vi "Process.vi"(8 "error in":errorcluster, 11 "Inst.Magneto":refnum<class "Inst.Magneto.lvclass">) -> (0 "error out":errorcluster, 3 "Inst.Magneto out":refnum<class "Inst.Magneto.lvclass">)   [LabVIEW 2019, in "Inst.Magneto.lvclass"]
doc: "---------------------------------------------------------------\nJKI State Machine Objects™\nhttp://jki.net/state-machine-objects/\nCopyright (C) 2005-2015, JKI <info@jki.net>\nALL RIGHTS RESERVED"
uses:
  Inst.Magneto.lvclass
  C:/Program Files (x86)/National Instruments/LabVIEW 2019/vi.lib/JKI/JKI SMO/SMO/SMO.lvclass
  C:/Program Files (x86)/National Instruments/LabVIEW 2019/user.lib/LevyLab/Instrument Framework/SMOs/Instrument/Instrument.lvclass
  Typedefs/Inst.Magneto.Commands--Enum.ctl
  Typedefs/PrivateEvents--Inst.Magneto.MessageToProcess.ctl
  <userlib>/LevyLab/Instrument Framework/SMOs/RemoteControl/Typedefs/Message--Cluster.ctl
  <vilib>/JKI/JKI SMO/SMO/SMO.lvclass/SMO.ctl
  Inst.Magneto.lvclass/Inst.Magneto.ctl
  <vilib>/JKI/JKI SMO/SMO/Private/ReftoDVR--SMO.vi
  <userlib>/LevyLab/Instrument Framework/Instrument Types/VSource/Instrument.VSource.lvclass
  <vilib>/JKI/JKI SMO/SMO/SMO.lvclass
  <userlib>/LevyLab/Instrument Framework/SMOs/Instrument/Instrument.lvclass
  <userlib>/LevyLab/Instrument Framework/SMOs/RemoteControl/RemoteControl.lvclass
  <vilib>/httpClient/LabVIEWHTTPClient.lvlib
panel:
  out "Status":string
  out "State History":string
  # "Instrument.Magneto"
  # "Magneto"
  # "For instructions on how to use the JKI State Machine Objects, examples and video tutorials, visit:\nhttp://jki.net/state-machine-objects/\n\nJKI State Machine Objects™\nhttp://jki.net/state-machine-objects/\nCopyright (C) 2005-2015, JKI <info@jki.net>\nALL RIGHTS RESERVED"
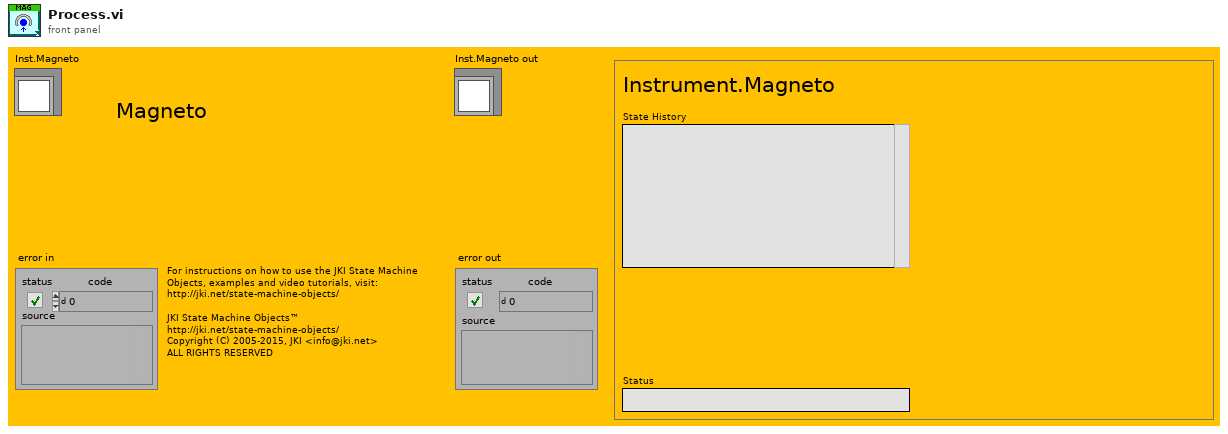
[diagram p1: front panel]
types:
  T1 = typedef "Inst.Magneto.lvclass/Inst.Magneto.Commands--Enum.ctl" = enum16{"GetRead", "Read", "Clear Values"}
  T2 = enum32{"invalid app kind", "Development System", "Run Time System", "Student Edition", "Embedded LabVIEW", "Evaluation", "Custom"}
  T3 = enum32{"Invalid", "Standard", "Closed", "Hidden", "Minimized", "Maximized"}
  T4 = typedef "RemoteControl.lvclass/Message--Cluster.ctl" = cluster{"Command":string, "Data":variant, "ID":string}
  T5 = typedef "Inst.Magneto.lvclass/PrivateEvents--Inst.Magneto.MessageToProcess.ctl" = cluster{"Message":T4}
  T6 = cluster{"Core":cluster{"Current VI Reference":refnum<vi>, "Close Panel on Exit?":bool, "Last Error":cluster{"error":errorcluster, "previous state":string, "remaining states":string}, "Shutdown?":bool}, "SelfRef":refnum<class "Inst.Magneto.lvclass">, "Running Step":i32, "sequence":string[], "MessageToProcess":T5}
  T7 = cluster{"Current VI Reference":refnum<vi>, "Close Panel on Exit?":bool, "Last Error":cluster{"error":errorcluster, "previous state":string, "remaining states":string}, "Shutdown?":bool}
  T8 = typedef "SMO.lvclass/Protected Events.ctl" = cluster{"StopProcesses":refnum<user-event>, "AbortProcesses":refnum<user-event>, "Config Changed":refnum<user-event>, "Dependency":refnum<user-event>}
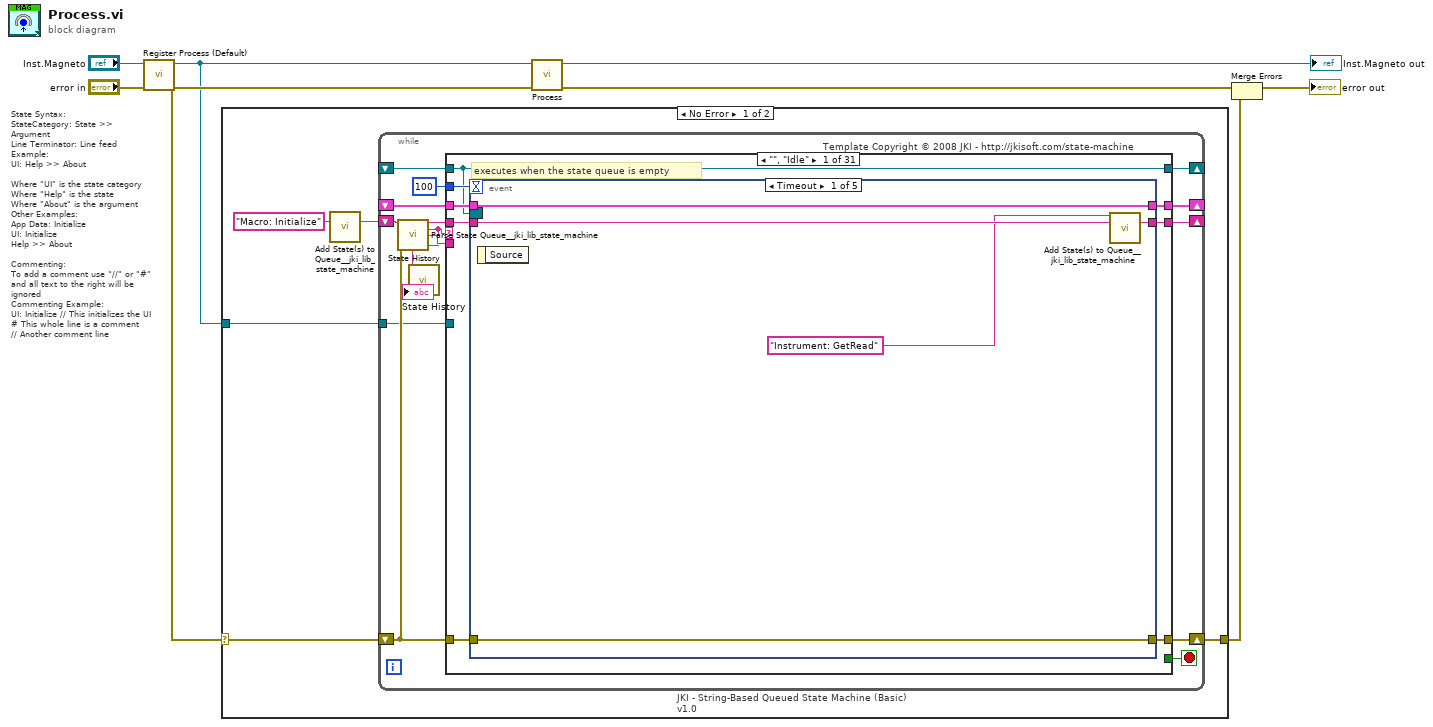
[diagram p0: block diagram]
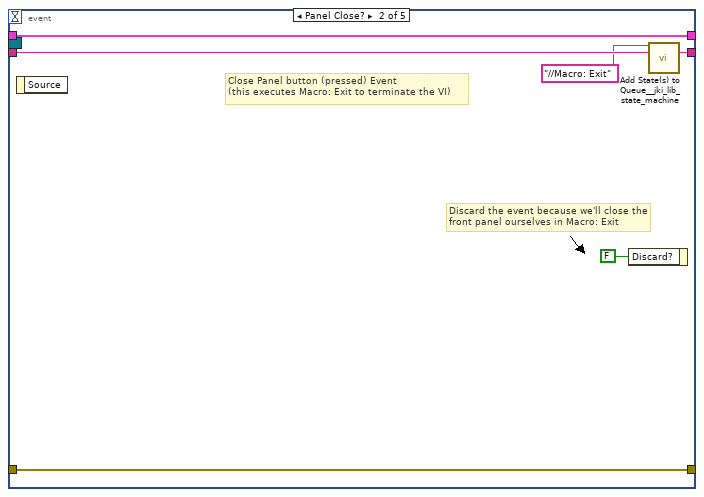
[diagram p2: hidden frame]
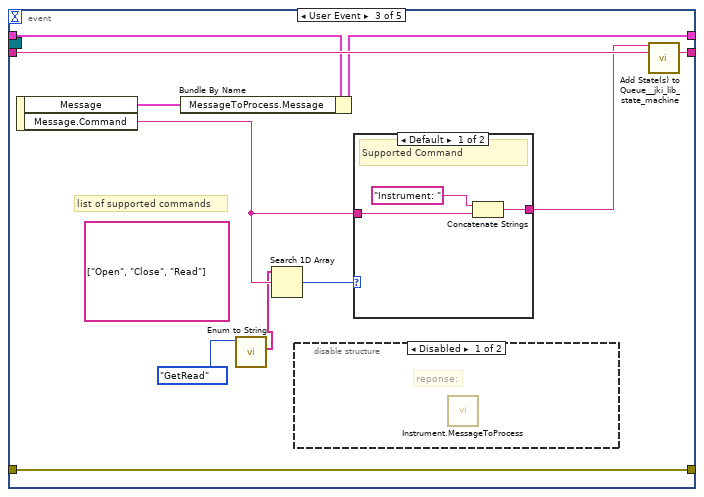
[diagram p3: hidden frame]
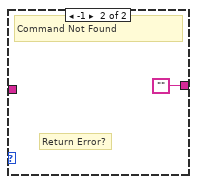
[diagram p5: hidden frame]
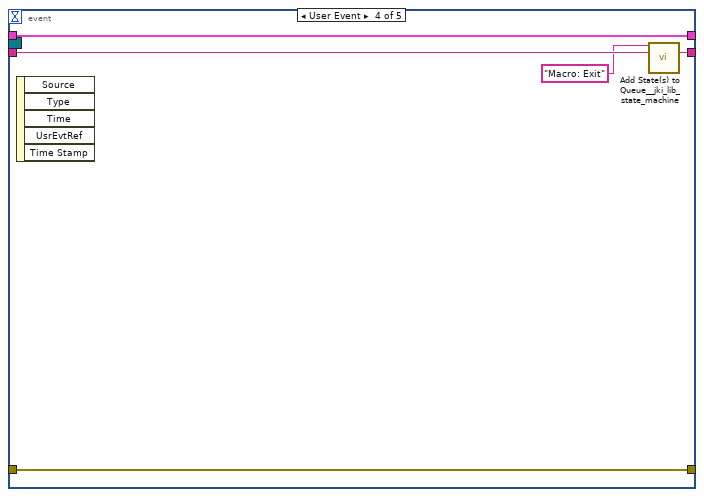
[diagram p6: hidden frame]
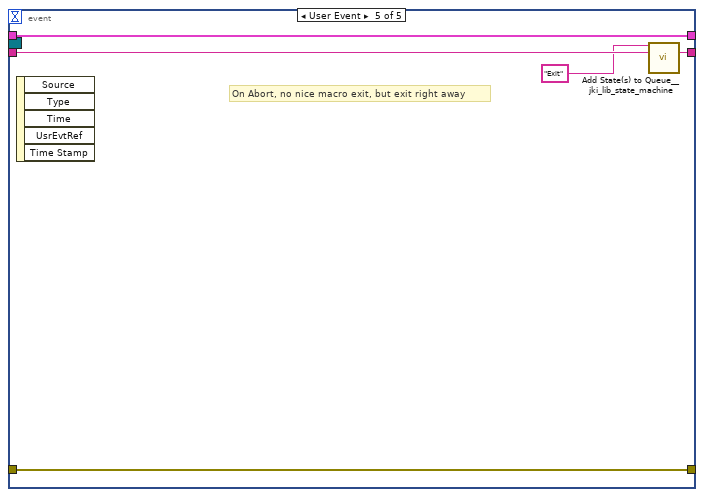
[diagram p7: hidden frame]
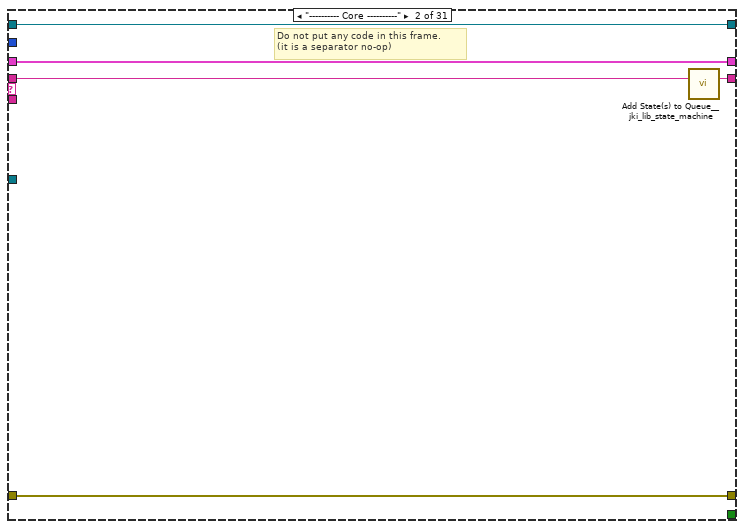
[diagram p8: hidden frame]
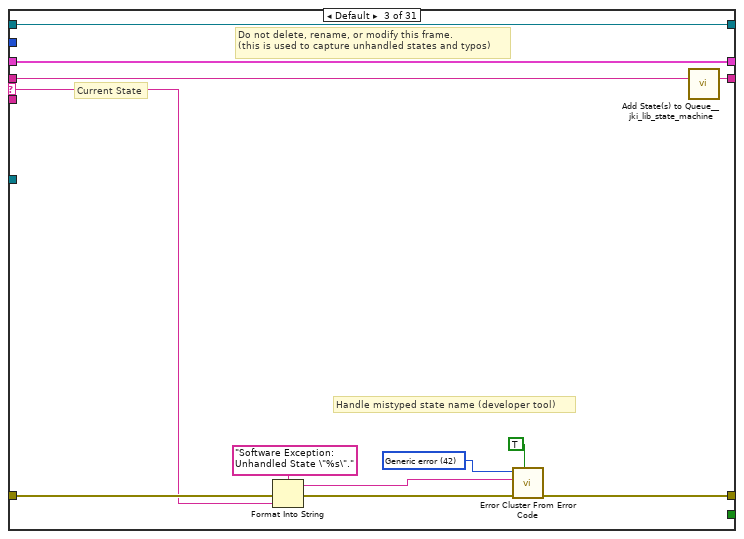
[diagram p9: hidden frame]
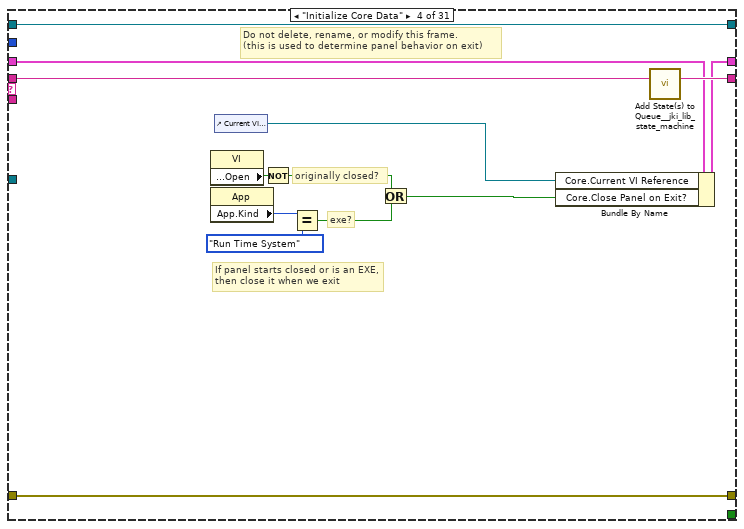
[diagram p10: hidden frame]
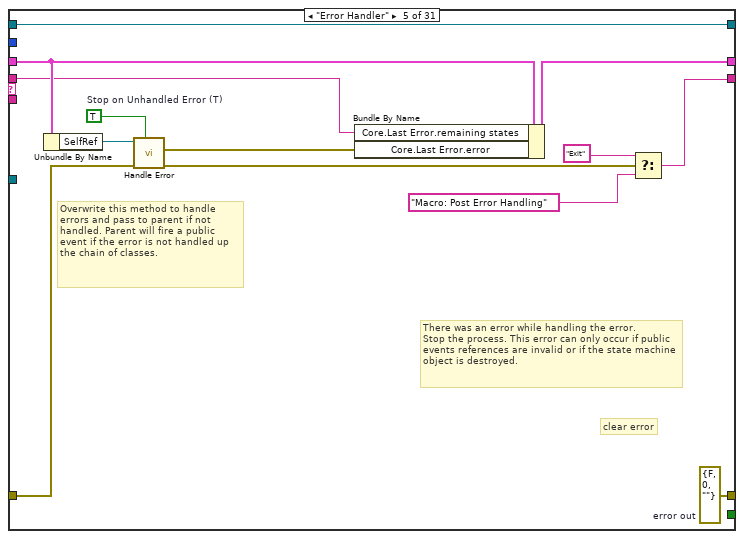
[diagram p11: hidden frame]
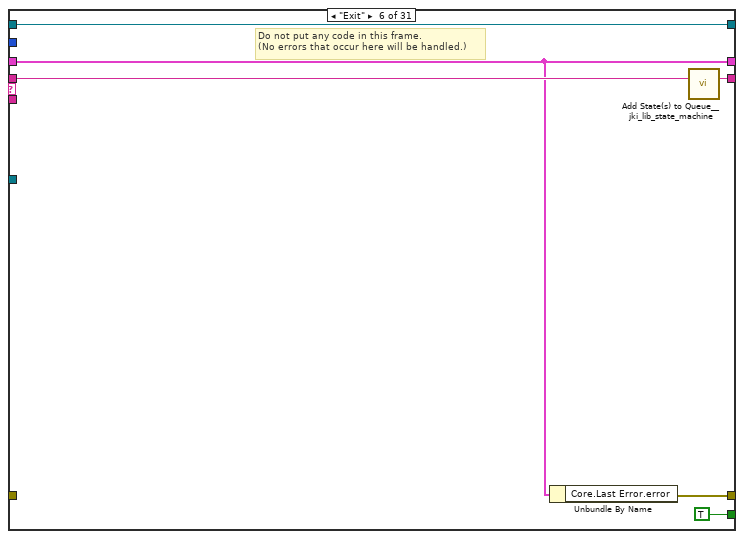
[diagram p12: hidden frame]
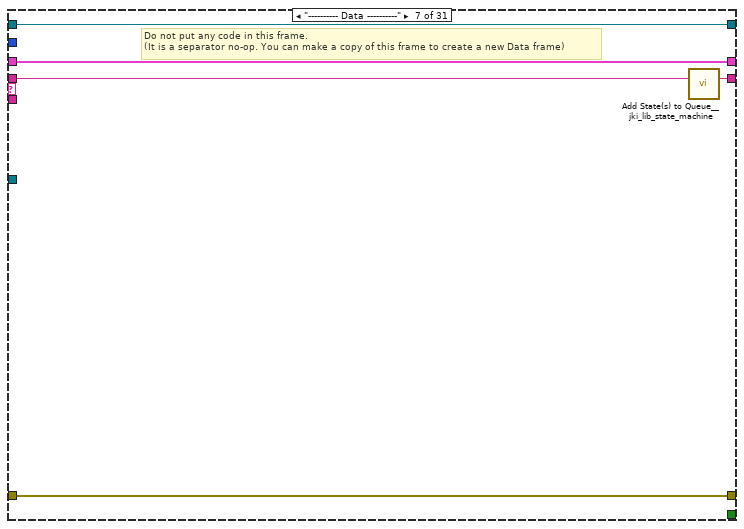
[diagram p13: hidden frame]
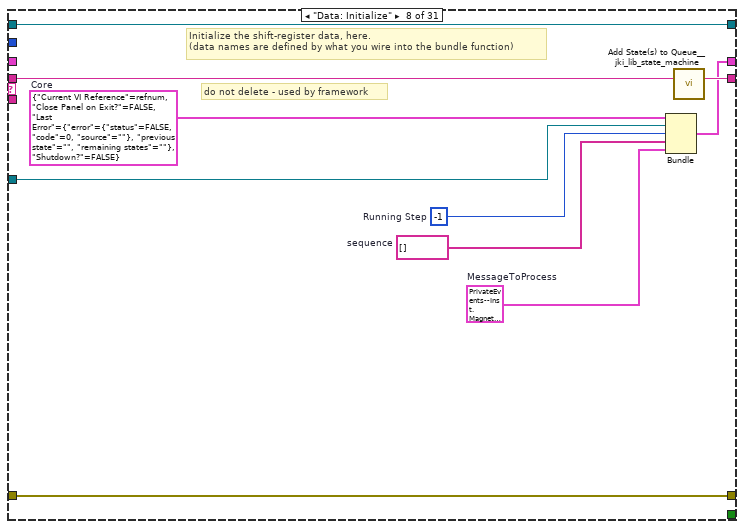
[diagram p14: hidden frame]
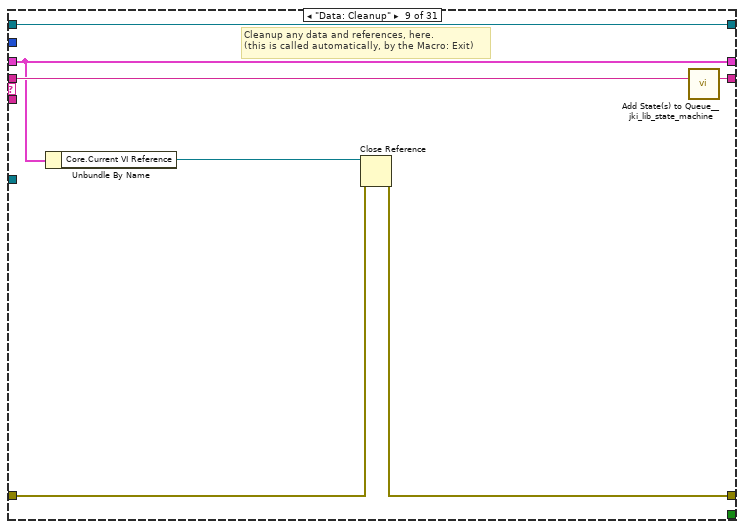
[diagram p15: hidden frame]
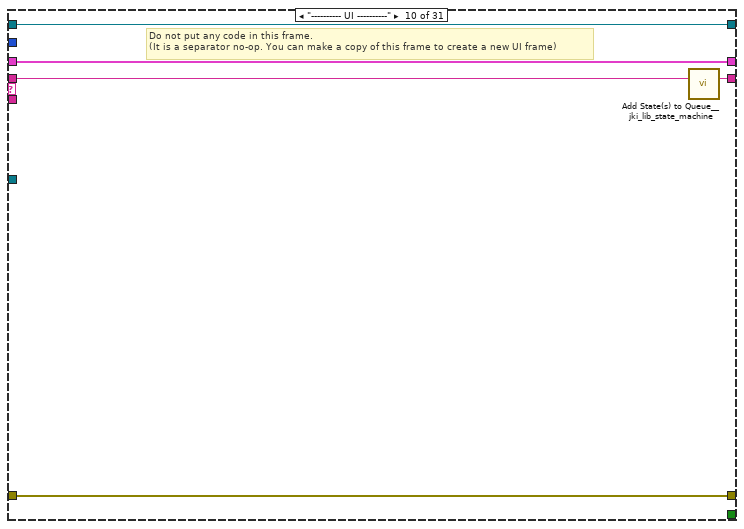
[diagram p16: hidden frame]
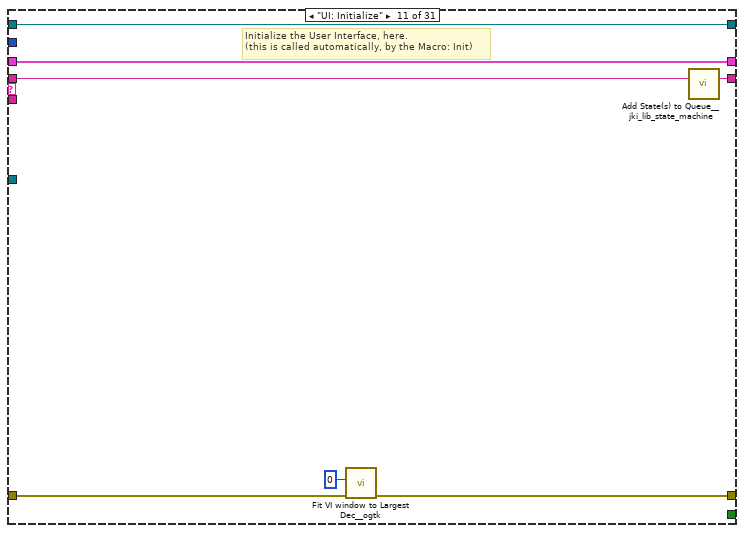
[diagram p17: hidden frame]
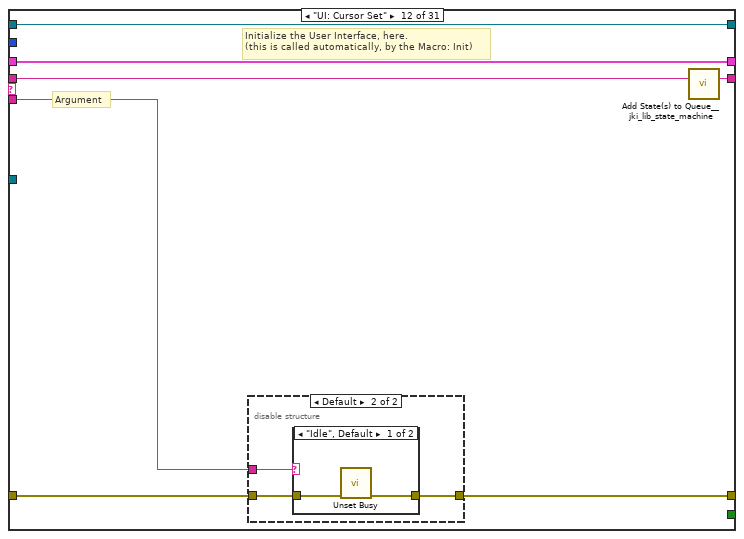
[diagram p18: hidden frame]
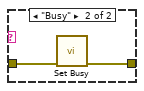
[diagram p20: hidden frame]
diagram:
  # "State Syntax:\nStateCategory: State >> Argument\nLine Terminator: Line feed\nExample:\nUI: Help >> About\n\nWhere \"UI\" is the state category\nWhere \"Help\" is the state\nWhere \"About\" is the argument\nOther Examples:\nApp Data: Initialize\nUI: Initialize\nHelp >> About\n\nCommenting:\nTo add a comment use \"//\" or \"#\" and all text to the right will be ignored\nCommenting Example:\nUI: Initialize // This initializes the UI\n# This whole line is a comment\n// Another comment line"
  n1 = call <vilib>:"Register Process (Default).vi"("error in (no error)"="error in", "SMO"="Inst.Magneto") -> ("error out"=w5:errorcluster, "SelfRef"=w4:refnum<class "Inst.Magneto.lvclass">)  [unwired: 8 in]
  n2 = case shown="No Error" w5 {
    selector: w5 -> [w10 w418]
    tunnel: w4 -> [w11 _]
    tunnel: [w9 w418] -> w1
    frame No Error {
      n3 = call <vilib>:"Add State(s) to Queue__jki_lib_state_machine.vi"("State(s) in (\"\")"="Macro: Initialize") -> ("States Out"=w13:string)  [unwired: 14 in]
      n4 = while "JKI - String-Based Queued State Machine (Basic) v1.0" {
        shift-right: [w22] -> _
        shift-left: _ -> [w21]
        shift-right: [w25] -> w9
        shift-left: w10 -> [w19]
        shift-right: [w24] -> _
        shift-left: w13 -> [w26]
        tunnel: w11 -> [w18]
        shift-right: [w17] -> _
        shift-left: _ -> [w16]
        stop <- w23 stop-if-true
        # "Template Copyright © 2008 JKI - http://jkisoft.com/state-machine"
        n5 = call <vilib>:"Parse State Queue__jki_lib_state_machine.vi"("State Queue"=w26, "Error In (no error)"=w19) -> ("Remaining States"=w28:string, "Current State"=w15:string, "Arguments"=w27:string)  [unwired: 11 in]
        n6 = call <userlib>:"State History.vi"("Current State"=w15) -> ("History"=→"State History":string)  [unwired: 10 in]
        n7 = case shown="\"\", \"Idle\"" w15 {
          selector: w15 -> [_ _ w79 _ _ _ _ _ _ _ _ _ _ _ _ _ _ _ _ _ _ _ _ _ _ _ _ _ _ _ _]
          tunnel: w28 -> [w36 w77 w83 w102 w107 w121 w126 w136 w143 w148 w155 w162 w178 w210 w229 w241 w262 w284 w289 w300 w305 w318 w324 w331 w340 w355 w364 w378 w392 w398 w417]
          tunnel: w27 -> [_ _ _ _ _ _ _ _ _ _ _ w156 w172 _ _ _ _ _ _ _ _ _ _ _ _ _ _ _ _ w393 w401]
          tunnel: w21 -> [w34 w74 w81 w93 w111 w117 w123 _ w138 w145 w153 w160 w174 w207 w226 w231 w252 w265 w286 w297 w302 w311 w322 w326 w336 w351 w360 w374 w388 w394 w407]
          tunnel: [w33 w75 w85 w99 w112 w116 w124 w128 w139 w146 w150 w157 w175 w208 w214 w239 w260 w267 w287 w291 w303 w314 w320 w328 w333 w349 w357 w369 w389 w395 w409] -> w25
          tunnel: w19 -> [w32 w75 w84 w99 w113 _ w124 w128 w140 w146 w149 w158 w176 w208 w218 w239 w260 w268 w287 w292 w303 w308 w320 w328 w332 w345 w356 w372 w389 w395 w403]
          tunnel: [w35 w76 w82 w101 w103 w120 w125 w135 w142 w147 w154 w161 w177 w209 w228 w240 w261 w283 w288 w299 w304 w317 w323 w330 w339 w354 w363 w377 w391 w397 w416] -> w24
          tunnel: [_ _ _ _ _ TRUE _ _ _ _ _ _ _ _ _ _ _ _ _ _ _ _ _ _ _ _ _ _ _ _ _] -> w23
          tunnel: [w31 w74 w81 w100 w110 w117 w123 w134 w138 w145 w153 w160 w174 w207 w226 w232 w253 w265 w286 w297 w302 w311 w322 w327 w337 w352 w361 w375 w388 w394 w406] -> w22
          tunnel: 100 ("Timeout") -> [w30 _ _ _ _ _ _ _ _ _ _ _ _ _ _ _ _ _ _ _ _ _ _ _ _ _ _ _ _ _ _]
          tunnel: w18 -> [_ _ _ _ _ _ _ w129 _ _ _ _ _ _ w222 _ _ w264 _ _ _ _ _ _ _ _ _ _ _ _ _]
          tunnel: [w29 w73 w78 w90 w115 w118 w122 w133 w137 w144 w152 w159 w171 w206 w227 w238 w259 w278 w285 w298 w301 w316 w321 w329 w338 w353 w362 w376 w390 w396 w415] -> w17
          tunnel: w16 -> [w29 w73 w78 w90 w115 w118 w122 w133 w137 w144 w152 w159 w171 w206 w227 w238 w259 w278 w285 w298 w301 _ w321 w329 w338 w353 w362 w376 w390 w396 w415]
          frame "", "Idle" {
            # "executes when the state queue is empty"
            n8 = event shown="[0] Timeout" {
              selector: w29 -> [_ _ _ _ _]
              dyn-events: _ -> [_ _ _ _ _]
              timeout: w30 -> [_ _ _ _ _]
              tunnel: w36 -> [w41 w47 w58 w67 w72]
              tunnel: [w40 w46 w57 w66 w71] -> w35
              tunnel: w34 -> [w38 w44 w51 w64 w69]
              tunnel: [w39 w45 w56 w65 w70] -> w33
              tunnel: w32 -> [w39 w45 w56 w65 w70]
              tunnel: [w38 w44 w52 w64 w69] -> w31
              event Timeout {
                n9 = event-data() -> ()  [unwired: 1 in, 1 out]
                n10 = call <vilib>:"Add State(s) to Queue__jki_lib_state_machine.vi"("State(s) in Front (\"\")"="Instrument: GetRead" ("State(s) in Front (\"\")"), "State(s) in (\"\")"=w41) -> ("States Out"=w40:string)  [unwired: 13 in]
              }
              event Panel Close? {
                # "Discard the event because we'll close the front panel ourselves in Macro: Exit"
                # "Close Panel button (pressed) Event\n(this executes Macro: Exit to terminate the VI)"
                n11 = event-data() -> ()  [unwired: 1 in, 1 out]
                n12 = event-data("Discard?"=FALSE) -> ()  [unwired: 1 in, 1 out]
                n13 = call <vilib>:"Add State(s) to Queue__jki_lib_state_machine.vi"("State(s) in Front (\"\")"="//Macro: Exit", "State(s) in (\"\")"=w47) -> ("States Out"=w46:string)  [unwired: 13 in]
              }
              event User Event {
                (unwired) string[] ["Open", "Close", "Read"]
                # "list of supported commands"
                n14 = event-data() -> ("Message"=w50:T4, "Message.Command"=w53:string)  [unwired: 1 in]
                n15 = Bundle By Name(cluster=w51, "MessageToProcess.Message"=w50) -> (w52:T6)
                n16 = call <userlib>:"Enum to String.vi"("Command"=Inst.Magneto.Commands--Enum."GetRead" ("Commands")) -> ("Commands []"=w48:string[])  [unwired: 9 in, 1 out]
                n17 = Search 1D Array(1D array=w48, element=w53) -> (index of element=w55:i32)  [unwired: 1 in]
                n18 = disable-structure shown="Disabled" {
                  frame Disabled {
                    # "reponse:"
                    n19 = call <userlib>:"Instrument.MessageToProcess.vi"() -> ()  [unwired: 10 in, 2 out]
                  }
                  frame Enabled {
                  }
                }
                n20 = case shown="Default" w55 {
                  tunnel: [w61 "" ("Empty String Constant")] -> w54
                  tunnel: w53 -> [w60 _]
                  frame Default {
                    # "Supported Command"
                    n21 = Concatenate Strings("Instrument: ", w60) -> (w61:string)
                  }
                  frame -1 {
                    # "Return Error?"
                    # "Command Not Found"
                  }
                }
                n22 = call <vilib>:"Add State(s) to Queue__jki_lib_state_machine.vi"("State(s) in Front (\"\")"=w54, "State(s) in (\"\")"=w58) -> ("States Out"=w57:string)  [unwired: 13 in]
              }
              event User Event {
                n23 = event-data() -> ()  [unwired: 1 in, 5 out]
                n24 = call <vilib>:"Add State(s) to Queue__jki_lib_state_machine.vi"("State(s) in Front (\"\")"="Macro: Exit", "State(s) in (\"\")"=w67) -> ("States Out"=w66:string)  [unwired: 13 in]
              }
              event User Event {
                # "On Abort, no nice macro exit, but exit right away"
                n25 = event-data() -> ()  [unwired: 1 in, 5 out]
                n26 = call <vilib>:"Add State(s) to Queue__jki_lib_state_machine.vi"("State(s) in Front (\"\")"="Exit", "State(s) in (\"\")"=w72) -> ("States Out"=w71:string)  [unwired: 13 in]
              }
            }
          }
          frame "---------- Core ----------" {
            # "Do not put any code in this frame.\n(it is a separator no-op)"
            n27 = call <vilib>:"Add State(s) to Queue__jki_lib_state_machine.vi"("State(s) in (\"\")"=w77) -> ("States Out"=w76:string)  [unwired: 14 in]
          }
          frame Default {
            w88 = 42 items=["No error", "Argument error", "Memory is full", "Out of zone", "End of file", "File already open", "Generic file I/O error", "File not found", "File permission error", "Disk is full", "Duplicate path", "Too many files open", "System feature not enabled", "Resource file not found", "Cannot add resource", "Resource not found", "Image not found", "Image memory error", "Pen does not exist", "Config type invalid", "Config token not found", "Config parse error", "Config memory error", "Bad external code format", "Bad external code offset", "External code not present", "Null window", "Destroy window error", "Null menu", "Print aborted", "Bad print record", "Print driver error", "Windows error during printing", "Memory error during printing", "Print dialog error", "Generic print error", "Invalid device refnum", "Device not found", "Device parameter error", "Device unit error", "Cannot open device", "Device call aborted", "Generic error", "Cancelled by user", "Object ID too low", "Object ID too high", "Object not in heap", "Unknown heap", "Unknown object (invalid DefProc)", "Unknown object (DefProc not in table)", "Message out of range", "Invalid (null) method", "Unknown message", "Manager call not supported", "Bad address", "Network operation in progress", "Network operation timed out", "Connection is busy", "Network attribute not supported", "Network error", "Address in use", "System out of memory", "Connection aborted", "Connection refused", "Not connected", "Already connected", "Connection closed", "Initialization error (interapplication manager)", "Bad occurrence", "Wait on unbound occurrence handler", "Occurrence queue overflow", "Datalog type conflict", "Unused", "Unrecognized type (interapplication manager)", "Memory corrupt", "Failed to make temporary DLL", "Old CIN version", "Drag socket not found", "Failed to load drop-object", "Failed to register OLE object", "Failed to release OLE object", "Format specifier type mismatch", "Unknown format specifier", "Too few format specifiers", "Too many format specifiers", "Scan failed", "Newer CIN version", "Error converting to variant", "Runtime menu error", "Password tampered", "Variant attribute not found", "Incompatible variant data type", "Event data is not available", "Event Store is not present", "Occurrence is not found", "Event Queue is not created", "Event info is not available", "Refnum passed is NULL", "Error retrieving Class GUID", "Error retrieving CoClass GUID", "Error retrieving TypeLib GUID.", "Bad built application magic bytes.", "Specific driver is different from the specific driver associated with the Logical Name.", "There is no session opened to the class driver.", "Max Error", "MAX - Error with config objects", "MAX - Error loading configuration", "MAX - Group not supported"]
            # "Current State"
            # "Do not delete, rename, or modify this frame.\n(this is used to capture unhandled states and typos)"
            # "Handle mistyped state name (developer tool)"
            n28 = Format Into String(format string="Software Exception: Unhandled State \"%s\"." ("message"), error in=w84, w79) -> (resulting string=w87:string, error out=w86:errorcluster)  [unwired: 1 in]
            n29 = call <vilib>:"Error Cluster From Error Code.vi"("show call chain? (False)"=TRUE, "error in (no error)"=w86, "error message (\"\")"=w87, "error code (0)"=w88) -> ("error out"=w85:errorcluster)  [unwired: 5 in]
            n30 = call <vilib>:"Add State(s) to Queue__jki_lib_state_machine.vi"("State(s) in (\"\")"=w83) -> ("States Out"=w82:string)  [unwired: 14 in]
          }
          frame "Initialize Core Data" {
            # "Do not delete, rename, or modify this frame.\n(this is used to determine panel behavior on exit)"
            # "originally closed?"
            # "exe?"
            # "If panel starts closed or is an EXE, then close it when we exit"
            n31 = property class="VI"() -> ("Front Panel.Open"=w98:bool)  [unwired: 2 in, 2 out]
            n32 = property class="App"() -> ("App.Kind"=w97:T2)  [unwired: 2 in, 2 out]
            n33 = control-ref of="Current VI Reference"() -> (w91:refnum<vi>)
            n34 = Not(x=w98) -> (.not. x?=w95:bool)
            n35 = Equal?(x=w97, y=T2."Run Time System" ("Application:Kind")) -> (x = y?=w94:bool)
            n36 = Or(x=w95, y=w94) -> (x .or. y?=w92:bool)
            n37 = Bundle By Name(cluster=w93, "Core.Current VI Reference"=w91, "Core.Close Panel on Exit?"=w92) -> (w100:T6)
            n38 = call <vilib>:"Add State(s) to Queue__jki_lib_state_machine.vi"("State(s) in (\"\")"=w102) -> ("States Out"=w101:string)  [unwired: 14 in]
          }
          frame "Error Handler" {
            w108 = TRUE  # Stop on Unhandled Error (T)
            w112 = errorcluster {"status"=FALSE, "code"=0, "source"=""}  # error out
            # "clear error"
            # "There was an error while handling the error.\nStop the process. This error can only occur if public events references are invalid or if the state machine object is destroyed."
            # "Overwrite this method to handle errors and pass to parent if not handled. Parent will fire a public event if the error is not handled up the chain of classes."
            n39 = Unbundle By Name(w111) -> ("SelfRef"=w114:refnum<class "Inst.Magneto.lvclass">)
            n40 = call-dynamic "Handle Error.vi"("Stop on Unhandled Error (T)"=w108, "error in"=w113, "SMO"=w114) -> ("handling error"=w104:errorcluster, "Unhandled error"=w109:errorcluster)  [unwired: 6 in, 1 out]
            n41 = Bundle By Name(cluster=w111, "Core.Last Error.remaining states"=w107, "Core.Last Error.error"=w109) -> (w110:T6)
            n42 = Select(t="Exit", s=w104, f="Macro: Post Error Handling") -> (s? t:f=w103:string)
          }
          frame "Exit" {
            # "Do not put any code in this frame.\n(No errors that occur here will be handled.)"
            n43 = Unbundle By Name(w117) -> ("Core.Last Error.error"=w116:errorcluster)
            n44 = call <vilib>:"Add State(s) to Queue__jki_lib_state_machine.vi"("State(s) in (\"\")"=w121) -> ("States Out"=w120:string)  [unwired: 14 in]
          }
          frame "---------- Data ----------" {
            # "Do not put any code in this frame.\n(It is a separator no-op. You can make a copy of this frame to create a new Data frame)"
            n45 = call <vilib>:"Add State(s) to Queue__jki_lib_state_machine.vi"("State(s) in (\"\")"=w126) -> ("States Out"=w125:string)  [unwired: 14 in]
          }
          frame "Data: Initialize" {
            w127 = T5 {"Message"={"Command"="", "Data"=variant(string ""), "ID"=""}}  # MessageToProcess
            w130 = string[] []  # sequence
            w131 = -1  # Running Step
            w132 = T7 {"Current VI Reference"=refnum, "Close Panel on Exit?"=FALSE, "Last Error"={"error"={"status"=FALSE, "code"=0, "source"=""}, "previous state"="", "remaining states"=""}, "Shutdown?"=FALSE}  # Core
            # "do not delete - used by framework"
            # "Initialize the shift-register data, here.\n(data names are defined by what you wire into the bundle function)"
            n46 = Bundle("Core"=w132, "SelfRef"=w129, "Running Step"=w131, "sequence"=w130, "MessageToProcess"=w127) -> (w134:T6)  [unwired: 1 in]
            n47 = call <vilib>:"Add State(s) to Queue__jki_lib_state_machine.vi"("State(s) in (\"\")"=w136) -> ("States Out"=w135:string)  [unwired: 14 in]
          }
          frame "Data: Cleanup" {
            # "Cleanup any data and references, here.\n(this is called automatically, by the Macro: Exit)"
            n48 = Unbundle By Name(w138) -> ("Core.Current VI Reference"=w141:refnum<vi>)
            n49 = Close Reference(reference=w141, error in (no error)=w140) -> (error out=w139:errorcluster)
            n50 = call <vilib>:"Add State(s) to Queue__jki_lib_state_machine.vi"("State(s) in (\"\")"=w143) -> ("States Out"=w142:string)  [unwired: 14 in]
          }
          frame "---------- UI ----------" {
            # "Do not put any code in this frame.\n(It is a separator no-op. You can make a copy of this frame to create a new UI frame)"
            n51 = call <vilib>:"Add State(s) to Queue__jki_lib_state_machine.vi"("State(s) in (\"\")"=w148) -> ("States Out"=w147:string)  [unwired: 14 in]
          }
          frame "UI: Initialize" {
            # "Initialize the User Interface, here.\n(this is called automatically, by the Macro: Init)"
            n52 = call <userlib>:"Fit VI window to Largest Dec__ogtk.vi"("error in (no error)"=w149, "border spacing (2 px)"=0) -> ("error out"=w150:errorcluster)  [unwired: 4 in, 1 out]
            n53 = call <vilib>:"Add State(s) to Queue__jki_lib_state_machine.vi"("State(s) in (\"\")"=w155) -> ("States Out"=w154:string)  [unwired: 14 in]
          }
          frame "UI: Cursor Set" {
            # "Argument"
            # "Initialize the User Interface, here.\n(this is called automatically, by the Macro: Init)"
            n54 = disable-structure shown="Default" {
              disable-tunnel: w158 -> [w163 w166]
              disable-tunnel: [w163 w165] -> w157
              disable-tunnel: w156 -> [_ w164]
              frame condition #0 {
              }
              frame condition #1 (active) {
                n55 = case shown="\"Idle\", Default" w164 {
                  tunnel: w166 -> [w168 w170]
                  tunnel: [w167 w169] -> w165
                  frame "Idle", Default {
                    n56 = call <vilib>:"Unset Busy.vi"("error in (no error)"=w168) -> ("error out"=w167:errorcluster)  [unwired: 10 in]
                  }
                  frame "Busy" {
                    n57 = call <vilib>:"Set Busy.vi"("error in (no error)"=w170) -> ("error out"=w169:errorcluster)  [unwired: 9 in, 1 out]
                  }
                }
              }
            }
            n58 = call <vilib>:"Add State(s) to Queue__jki_lib_state_machine.vi"("State(s) in (\"\")"=w162) -> ("States Out"=w161:string)  [unwired: 14 in]
          }
          frame "UI: Front Panel State" {
            # "Argument"
            # "Set Front Panel Open or Closed\n(Usage: \"UI: Front Panel State >> Open|Close\")"
            n59 = Unbundle By Name(w174) -> ("Core.Current VI Reference"=w173:refnum<vi>)
            n60 = disable-structure shown="Default" {
              disable-tunnel: w176 -> [w182 w205]
              disable-tunnel: [w181 w205] -> w175
              disable-tunnel: w173 -> [w180 _]
              disable-tunnel: w172 -> [w179 _]
              frame condition #0 (active) {
                n61 = case shown="\"Close\"" w179 {
                  tunnel: w182 -> [w186 w199]
                  tunnel: [w188 w200] -> w181
                  tunnel: w180 -> [w187 w197]
                  frame "Open", Default {
                    n62 = property class="VI"(reference=w187, error in=w186) -> (reference out=w184:refnum<vi>, error out=w185:errorcluster, "FP.State"=w183:T3)
                    n63 = case shown="\"Closed\"" w183 {
                      tunnel: [w191 w194] -> w188
                      tunnel: w185 -> [w190 w194]
                      tunnel: w184 -> [w189 _]
                      frame "Closed" {
                        n64 = invoke class="VI" method="FP.Open"(reference=w189, error in=w190, "Activate"=TRUE, "State"=T3."Standard") -> (error out=w191:errorcluster)  [unwired: 1 in, 4 out]
                      }
                      frame Default {
                      }
                    }
                  }
                  frame "Close" {
                    n65 = property class="VI"(reference=w197, error in=w199) -> (reference out=w196:refnum<vi>, error out=w198:errorcluster, "FP.State"=w195:T3)
                    n66 = case shown="Default" w195 {
                      tunnel: [w201 w204] -> w200
                      tunnel: w198 -> [w201 w203]
                      tunnel: w196 -> [_ w202]
                      frame "Invalid", "Closed" {
                      }
                      frame Default {
                        n67 = invoke class="VI" method="FP.Close"(reference=w202, error in=w203) -> (error out=w204:errorcluster)  [unwired: 1 in, 2 out]
                      }
                    }
                  }
                }
              }
              frame condition #1 {
              }
            }
            n68 = call <vilib>:"Add State(s) to Queue__jki_lib_state_machine.vi"("State(s) in (\"\")"=w178) -> ("States Out"=w177:string)  [unwired: 14 in]
          }
          frame "---------- Macro ----------" {
            # "Do not put any code in this frame.\n(It is a separator no-op. You can make a copy of this frame to create a new Macro frame)"
            n69 = call <vilib>:"Add State(s) to Queue__jki_lib_state_machine.vi"("State(s) in (\"\")"=w210) -> ("States Out"=w209:string)  [unwired: 14 in]
          }
          frame "Macro: Initialize" {
            # "Initialization Macro\n(This is called once, when the VI starts)"
            n70 = call-dynamic "Read Debug Mode.vi"("error in (no error)"=w218, "Instrument in"=w222) -> ("error out"=w217:errorcluster, "Debug Mode?"=w219:bool)  [unwired: 7 in, 1 out]
            n71 = call <userlib>:"Wait (ms)__ogtk.vi"("error in (no error)"=w217, "milliseconds to wait"=u32 0) -> ("error out"=w214:errorcluster)  [unwired: 8 in, 1 out]
            n72 = Select(t="Open", s=w219, f="Close") -> (s? t:f=w215:string)
            n73 = Format Into String(format string="UI: Initialize\nUI: Front Panel State >> %s\nInstrument: Open Hardware", initial string="", w215) -> (resulting string=w216:string)  [unwired: 1 in, 1 out]
            n74 = call <vilib>:"Add State(s) to Queue__jki_lib_state_machine.vi"("State(s) in Front (\"\")"="Data: Initialize\nInitialize Core Data\nEvents: Register", "State(s) in (\"\")"="Process: Sync", "State(s) at Back (\"\")"=w216) -> ("States Out"=w224:string)  [unwired: 12 in]
            n75 = call <vilib>:"Add State(s) to Queue__jki_lib_state_machine.vi"("State(s) in Front (\"\")"=w224, "State(s) in (\"\")"=w229) -> ("States Out"=w228:string)  [unwired: 13 in]
          }
          frame "Macro: Post Error Handling" {
            # "Clear Last Error?"
            n76 = Unbundle By Name(w231) -> ("Core.Last Error.remaining states"=w233:string, "Core.Shutdown?"=w234:bool)
            n77 = Unbundle By Name(w231) -> ("Core.Last Error.error"=w237:errorcluster)
            n78 = case shown="False" FALSE {
              tunnel: w237 -> [w245 _]
              tunnel: [w245 _] -> w236
              frame False {
              }
              frame True {
              }
            }
            n79 = case shown="True" w234 {
              tunnel: w233 -> [w242 w244]
              tunnel: [w242 w243] -> w230
              frame False {
                # "These are the remaining states (at the moment the error occured). States can be altered according to business logic."
                # "NOT SHUTTING DOWN"
              }
              frame True {
                # "Developer can decide to alter the states but should be aware that during the shutdown process, there are certain states that must be run for the SMO to properly shut itself (and this process) down. As such, one can add states to perform additional clean-ups, but should append the remaining state to be executed."
                # "SHUTTING DOWN"
                n80 = call <vilib>:"Add State(s) to Queue__jki_lib_state_machine.vi"("State(s) in (\"\")"=w244) -> ("States Out"=w243:string)  [unwired: 14 in]
              }
            }
            n81 = Bundle By Name(cluster=w231, "Core.Last Error.error"=w236) -> (w232:T6)
            n82 = call <vilib>:"Add State(s) to Queue__jki_lib_state_machine.vi"("State(s) in Front (\"\")"=w230, "State(s) in (\"\")"=w241) -> ("States Out"=w240:string)  [unwired: 13 in]
          }
          frame "Macro: Run Sequence" {
            # "0,1,2,3,4,"
            # "5"
            # "Do not put any code in this frame.\n(It is a separator no-op. You can make a copy of this frame to create a new Macro frame)"
            n83 = Unbundle By Name(w252) -> ("sequence"=w248:string[], "Running Step"=w246:i32)
            n84 = Array Size(array=w248) -> (size(s)=w258:i32)
            n85 = Index Array(array=w248, index=w246) -> (element=w247:string)
            n86 = Greater Or Equal?(x=w258, y=w246) -> (x >= y?=w250:bool)
            n87 = Select(t=-1 ("Running Step"), s=w250, f=w246) -> (s? t:f=w257:i32)
            n88 = Bundle By Name(cluster=w252, "Running Step"=w257) -> (w253:T6)
            n89 = Select(t="Sequence: Status >> ...", s=w250, f="Idle //Check Event Structure\nMacro: Run Sequence" ("State(s) at Back (\"\")")) -> (s? t:f=w249:string)
            n90 = call <vilib>:"Add State(s) to Queue__jki_lib_state_machine.vi"("State(s) in Front (\"\")"=w247, "State(s) at Back (\"\")"=w249) -> ("States Out"=w251:string)  [unwired: 13 in]
            n91 = call <vilib>:"Add State(s) to Queue__jki_lib_state_machine.vi"("State(s) in Front (\"\")"=w251, "State(s) in (\"\")"=w262) -> ("States Out"=w261:string)  [unwired: 13 in]
          }
          frame "Macro: Exit" {
            # "Exit Macro\n(This is called once, when the VI exits)"
            n92 = Unbundle By Name(w265) -> ("Core.Close Panel on Exit?"=w282:bool)
            n93 = call-dynamic "Read Debug Mode.vi"("error in (no error)"=w268, "Instrument in"=w264) -> ("error out"=w267:errorcluster, "Debug Mode?"=w266:bool)  [unwired: 7 in, 1 out]
            n94 = Select(t="Open", s=w266, f="Close") -> (s? t:f=w272:string)
            n95 = call <vilib>:"Build State String with Arguments__JKI_lib_State_Machine.vi"("Arguments (\"\")"=w272, "State"="UI: Front Panel State") -> ("State with Arguments"=w269:string)  [unwired: 4 in]
            n96 = Select(t=w269, s=w282, f="" ("Empty String Constant")) -> (s? t:f=w280:string)
            n97 = call <vilib>:"Add State(s) to Queue__jki_lib_state_machine.vi"("State(s) in Front (\"\")"="Data: Cleanup\nEvents: Unregister", "State(s) in (\"\")"="Process: Sync", "State(s) at Back (\"\")"="Exit") -> ("States Out"=w275:string)  [unwired: 12 in]
            n98 = call <vilib>:"Add State(s) to Queue__jki_lib_state_machine.vi"("State(s) in Front (\"\")"="Instrument: Close Hardware", "State(s) in (\"\")"=w280, "State(s) at Back (\"\")"=w275) -> ("States Out"=w279:string)  [unwired: 12 in]
            n99 = call <vilib>:"Add State(s) to Queue__jki_lib_state_machine.vi"("State(s) in Front (\"\")"=w279, "State(s) in (\"\")"=w284) -> ("States Out"=w283:string)  [unwired: 13 in]
          }
          frame "---------- Process ----------" {
            # "Template Separator\n(You can make a copy of, or modify, this frame)"
            n100 = call <vilib>:"Add State(s) to Queue__jki_lib_state_machine.vi"("State(s) in (\"\")"=w289) -> ("States Out"=w288:string)  [unwired: 14 in]
          }
          frame "Process: Sync" {
            n101 = Unbundle By Name(w297) -> ("SelfRef"=w293:refnum<class "Inst.Magneto.lvclass">)
            n102 = call <vilib>:"WaitOnProcessSync.vi"("error in (no error)"=w292, "SMO"=w293) -> ("error out"=w291:errorcluster, "Don't run?"=w296:bool)  [unwired: 7 in, 1 out]
            n103 = Select(t="Data: Cleanup\nEvents: Unregister\nExit", s=w296, f="" ("Empty String Constant")) -> (s? t:f=w290:string)
            n104 = call <vilib>:"Add State(s) to Queue__jki_lib_state_machine.vi"("State(s) in Front (\"\")"=w290, "State(s) in (\"\")"=w300) -> ("States Out"=w299:string)  [unwired: 13 in]
          }
          frame "---------- Events ----------" {
            # "Template Separator\n(You can make a copy of, or modify, this frame)"
            n105 = call <vilib>:"Add State(s) to Queue__jki_lib_state_machine.vi"("State(s) in (\"\")"=w305) -> ("States Out"=w304:string)  [unwired: 14 in]
          }
          frame "Events: Register" {
            n106 = Unbundle By Name(w311) -> ("SelfRef"=w312:refnum<class "Inst.Magneto.lvclass">)
            n107 = call <vilib>:"GetProtectedEvents.vi"("SMO"=w312) -> ("error out"=w310:errorcluster, "SMO Protected Events"=w315:T8, "SMO out"=w309:refnum<class "Inst.Magneto.lvclass">)  [unwired: 8 in]
            n108 = call "Inst.Magneto.GetPrivateEvents.vi"("Inst.Magneto in"=w309) -> ("error out"=w306:errorcluster, "Inst.Magneto Private Events"=w307:cluster{"MessageToProcess":refnum<user-event>})  [unwired: 8 in, 1 out]
            n109 = register-events(w315, w307) -> (reference out=w316:refnum<event-registration>, error out=w313:errorcluster)  [unwired: 2 in]
            n110 = Merge Errors(w313, w306, w310, w308) -> (w314:errorcluster)
            n111 = call <vilib>:"Add State(s) to Queue__jki_lib_state_machine.vi"("State(s) in (\"\")"=w318) -> ("States Out"=w317:string)  [unwired: 14 in]
          }
          frame "Events: Unregister" {
            n112 = Unregister For Events(event registration refnum=w321, error in=w320) -> (error out=w319:errorcluster)
            n113 = call <vilib>:"Clear Errors.vi"("error in (no error)"=w319) -> ()  [unwired: 5 in, 2 out]
            n114 = call <vilib>:"Add State(s) to Queue__jki_lib_state_machine.vi"("State(s) in (\"\")"=w324) -> ("States Out"=w323:string)  [unwired: 14 in]
          }
          frame "---------- Instrument ----------" {
            n115 = Unbundle By Name(w326) -> ("SelfRef"=w325:refnum<class "Inst.Magneto.lvclass">)
            n116 = Bundle By Name(cluster=w326, "SelfRef"=w325) -> (w327:T6)
            n117 = call <vilib>:"Add State(s) to Queue__jki_lib_state_machine.vi"("State(s) in (\"\")"=w331) -> ("States Out"=w330:string)  [unwired: 14 in]
          }
          frame "Instrument: Open Hardware" {
            n118 = Unbundle By Name(w336) -> ("SelfRef"=w335:refnum<class "Inst.Magneto.lvclass">)
            n119 = call-dynamic "Open Hardware.vi"("error in (no error)"=w332, "Inst.Magneto in"=w335) -> ("error out"=w333:errorcluster, "Inst.Magneto out"=w334:refnum<class "Inst.Magneto.lvclass">)  [unwired: 8 in]
            n120 = Bundle By Name(cluster=w336, "SelfRef"=w334) -> (w337:T6)
            n121 = call <vilib>:"Add State(s) to Queue__jki_lib_state_machine.vi"("State(s) in (\"\")"=w340) -> ("States Out"=w339:string)  [unwired: 14 in]
          }
          frame "Instrument: GetRead" {
            w347 = "http://10.226.177.141:5000/sensors"  # Server Address
            # "send data to\ninstrument:process.vi"
            n122 = Unbundle By Name(w351) -> ("SelfRef"=w341:refnum<class "Inst.Magneto.lvclass">, "MessageToProcess.Message.ID"=w348:string)
            n123 = call <vilib>:"GET.vi"("url"=w347, "error in (no error)"=w345) -> ("body"=w343:string, "error out"=w346:errorcluster)  [unwired: 10 in, 2 out]
            n124 = To Variant(anything=w343) -> (Variant=w342:variant)
            n125 = call <userlib>:"Instrument.MessageToProcess.vi"("ID"=w348, "error in (no error)"=w346, "Data"=w342, "Command"="Read", "Instrument"=w341) -> ("error out"=w349:errorcluster, "Instrument out"=w350:refnum<class "Inst.Magneto.lvclass">)  [unwired: 5 in]
            n126 = Bundle By Name(cluster=w351, "SelfRef"=w350) -> (w352:T6)
            n127 = call <vilib>:"Add State(s) to Queue__jki_lib_state_machine.vi"("State(s) in (\"\")"=w355) -> ("States Out"=w354:string)  [unwired: 14 in]
          }
          frame "Instrument: Close Hardware" {
            n128 = Unbundle By Name(w360) -> ("SelfRef"=w359:refnum<class "Inst.Magneto.lvclass">)
            n129 = call-dynamic "Close Hardware.vi"("error in (no error)"=w356, "Inst.Magneto in"=w359) -> ("error out"=w357:errorcluster, "Inst.Magneto out"=w358:refnum<class "Inst.Magneto.lvclass">)  [unwired: 8 in]
            n130 = Bundle By Name(cluster=w360, "SelfRef"=w358) -> (w361:T6)
            n131 = call <vilib>:"Add State(s) to Queue__jki_lib_state_machine.vi"("State(s) in (\"\")"=w364) -> ("States Out"=w363:string)  [unwired: 14 in]
          }
          frame "Instrument: GetAll" {
            # "communicate with\nhardware"
            n132 = Unbundle By Name(w374) -> ("SelfRef"=w373:refnum<class "Inst.Magneto.lvclass">, "MessageToProcess.Message.ID"=w365:string)
            n133 = call "Inst.Magneto.DoSomething.vi"("error in (no error)"=w372, "Inst.Magneto in"=w373) -> ("error out"=w368:errorcluster, "Data out"=w367:variant, "Inst.Magneto out"=w371:refnum<class "Inst.Magneto.lvclass">)  [unwired: 7 in]
            n134 = Empty String/Path?(string/path=w367) -> (empty?=w366:bool)
            n135 = case shown="False" w366 {
              tunnel: w371 -> [w385 w387]
              tunnel: [w384 w387] -> w370
              tunnel: [w383 w386] -> w369
              tunnel: w367 -> [w380 _]
              tunnel: w368 -> [w379 w386]
              tunnel: w365 -> [w381 _]
              frame False {
                # "send data to\ninstrument:process.vi"
                n136 = call <userlib>:"Instrument.MessageToProcess.vi"("ID"=w381, "error in (no error)"=w379, "Data"=w380, "Command"="Set GetAll", "Instrument"=w385) -> ("error out"=w383:errorcluster, "Instrument out"=w384:refnum<class "Inst.Magneto.lvclass">)  [unwired: 5 in]
              }
              frame True {
              }
            }
            n137 = Bundle By Name(cluster=w374, "SelfRef"=w370) -> (w375:T6)
            n138 = call <vilib>:"Add State(s) to Queue__jki_lib_state_machine.vi"("State(s) in (\"\")"=w378) -> ("States Out"=w377:string)  [unwired: 14 in]
          }
          frame "---------- Sequence ----------" {
            n139 = call <vilib>:"Add State(s) to Queue__jki_lib_state_machine.vi"("State(s) in (\"\")"=w392) -> ("States Out"=w391:string)  [unwired: 14 in]
          }
          frame "Sequence: Status" {
            # "Sequence: Status\n(Use this frame to pass the status to the UI, this VI's UI, etc)"
            n140 = call <vilib>:"Add State(s) to Queue__jki_lib_state_machine.vi"("State(s) in (\"\")"=w398) -> ("States Out"=w397:string)  [unwired: 14 in]
            "Status" <- w393
          }
          frame "Sequence: Wait" {
            # "Sequence: Wait\n(Non-Blocking Wait)"
            # "F = repeat this state. wait\nT = go to next state. don't wait"
            n141 = Unbundle By Name(w407) -> ("Running Step"=w400:i32)
            n142 = call <userlib>:"Wait Logic.vi"("error in (no error)"=w403, "Time"=w401) -> ("error out"=w402:errorcluster, "Status String"=w399:string, "Trigger"=w404:bool)  [unwired: 6 in, 1 out]
            n143 = Increment(x=w400) -> (x+1=w414:i32)
            n144 = Select(t=w414, s=w404, f=w400) -> (s? t:f=w405:i32)
            n145 = Select(t=u32 0, s=w404, f=u32 100 ("milliseconds to wait")) -> (s? t:f=w411:u32)
            n146 = call <userlib>:"Wait (ms)__ogtk.vi"("error in (no error)"=w402, "milliseconds to wait"=w411) -> ("error out"=w409:errorcluster)  [unwired: 8 in, 1 out]
            n147 = Bundle By Name(cluster=w407, "Running Step"=w405) -> (w406:T6)
            n148 = call <vilib>:"Build State String with Arguments__JKI_lib_State_Machine.vi"("Arguments (\"\")"=w399, "State"="Sequence: Status") -> ("State with Arguments"=w408:string)  [unwired: 4 in]
            n149 = call <vilib>:"Add State(s) to Queue__jki_lib_state_machine.vi"("State(s) in Front (\"\")"=w408, "State(s) in (\"\")"=w417) -> ("States Out"=w416:string)  [unwired: 13 in]
          }
        }
      }
    }
    frame Error {
    }
  }
  n150 = call-parent "Process.vi"("error in"=w5, "Instrument"=w4) -> ("error out"=w2:errorcluster, "Instrument out"=→"Inst.Magneto out":refnum<class "Inst.Magneto.lvclass">)  [unwired: 8 in]
  n151 = Merge Errors(w2, w1) -> (→"error out":errorcluster)
